vi "MM9.SetStatus.vi"(0 "i ref in":refnum<vi>, 1 "MMStatusSuccess":T1, 2 "MMStatusFail":T1, 3 "ms timeout (10000)":i32=10000, 5 "error in (no error)":errorcluster) -> (14 "i ref out":refnum<vi>, 16 "StatusText":string, 17 "timed out":bool, 19 "error out":errorcluster)   [LabVIEW 2014, in "MM9.lvlib"]
doc: "Sets the status of the measurement."
uses:
  MM9.lvlib
  MM9.status.ctl
  CS_Core/CSSystem/CoreLib/CoreLib.lvlib
  CSlibraries-extern/DimLVEvent/LVDimInterface/LVDimInterface.lvlib
panel:
  in  "MMStatus":T1=enum."config"
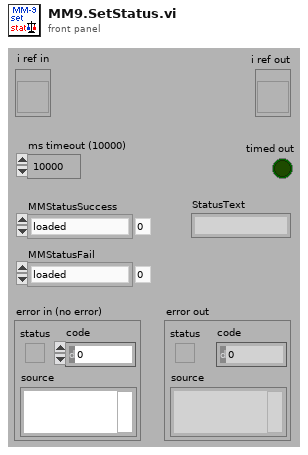
[diagram p1: front panel]
types:
  T1 = typedef "MM9.lvlib/MM9.status.ctl" = enum16{"loaded", "load_error", "config", "config_error", "init", "init_error", "data_reset", "data_reset_error", "running", "start_error", "run_error", "abort_requested", "aborted", "stop_requested", "stopped", "stop_error", "Connected", "NOTConnected"}
  T2 = typedef "MM9.lvlib/MM9.i attribute.ctl" = cluster{"UsedObjs":string[], "ActScanStep":i32[], "AbortRequest":bool, "StopRequest":bool, "# cycles":i32, "Connected":bool, "MMStatus":T1, "# data":i32, "DIMServices":cluster{"MM6StatusString":string, "MM6StatusID":i32, "discArchiver":string, "discArchiverID":i32, "eventBuilder":string, "eventBuilderID":i32, "GUIIDString":string, "GUIIDStringID":i32}, "dataFile":string, "PGRunning":T3, "ConfigData":T4, "ExtraDataSets":T19}
  T3 = typedef "PPG_ABC.lvlib/PPG_ABC.PG_Running.ctl" = i32
  T4 = typedef "LEBITDefs9.lvlib/LEBITDefs.ConfigData.ctl" = cluster{"GenConfig":T5, "Configs":T7[]}
  T5 = typedef "LEBITDefs9.lvlib/LEBITDefs.GenConfig.ctl" = cluster{"Mode":i32, "Logs":T6[]}
  T6 = typedef "LEBITDefs9.lvlib/LEBITDefs.Log.ctl" = cluster{"Name":string, "FctName":string, "Special":string}
  T7 = typedef "LEBITDefs9.lvlib/LEBITDefs.OneConfig.ctl" = cluster{"MCA":T8, "Timing":T9, "Scans":T12[], "FreqDevs":T13[], "CleanDev":T14, "NrCycles":i32, "Specials":T16[], "Delays":T17[], "DAC":T18}
  T8 = typedef "LEBITDefs9.lvlib/LEBITDefs.MCA.ctl" = cluster{"Name":string, "Address":string, "NrChannels":i32, "Gate":i32, "NrPipse":i32, "AcqDelay":i32}
  T9 = typedef "LEBITDefs9.lvlib/LEBITDefs.Timing.ctl" = cluster{"TimeTables":cluster{"TimeTable":T10}[], "Memories":T11[], "ScanX":string, "ScanY":string}
  T10 = typedef "LEBITDefs9.lvlib/LEBITDefs.Timetable.ctl" = dbl[]
  T11 = typedef "LEBITDefs9.lvlib/LEBITDefs.Memory.ctl" = cluster{"Device":string, "ExtTrig":bool, "TT2Use":i32, "PatternTable":string[]}
  T12 = typedef "LEBITDefs9.lvlib/LEBITDefs.ScanDev.ctl" = cluster{"Name":string, "FctName":string, "Values":dbl[], "NrScanVals":i32, "Special":string}
  T13 = typedef "LEBITDefs9.lvlib/LEBITDefs.FreqDev.ctl" = cluster{"Name":string, "Amp":dbl, "CenterFreq":dbl, "Time":dbl}
  T14 = typedef "LEBITDefs9.lvlib/LEBITDefs.CleanDev.ctl" = cluster{"Name":string, "CleanData":T15[]}
  T15 = typedef "LEBITDefs9.lvlib/LEBITDefs.CleanDataType.ctl" = cluster{"Amp":dbl, "Center":dbl, "Plus":dbl, "Minus":dbl, "Time":dbl}
  T16 = typedef "LEBITDefs9.lvlib/LEBITDefs.Special.ctl" = cluster{"Name":string, "FctName":string, "VerySpecial":string, "Data":dbl}
  T17 = typedef "LEBITDefs9.lvlib/LEBITDefs.Delay.ctl" = cluster{"Name":string, "Delay":dbl}
  T18 = typedef "LEBITDefs9.lvlib/LEBITDefs.DAC.ctl" = cluster{"Name":string, "Step1":i32, "Step2":i32}
  T19 = typedef "LEBITDefs9.lvlib/LEBITDefs.ExtraData.ctl" = cluster{"Ions":cluster{"ExcitIonMass":string, "ExcitIonCharge":i32, "CleanIons":cluster{"CleanIonMass":string, "CleanIonCharge":i32}[]}, "TimingDescription":cluster{"TimeTableDescription":cluster{"Times":string[]}[], "PatternTableDescription":cluster{"Pattern":string[]}[]}, "ScanUnits":string[]}[]
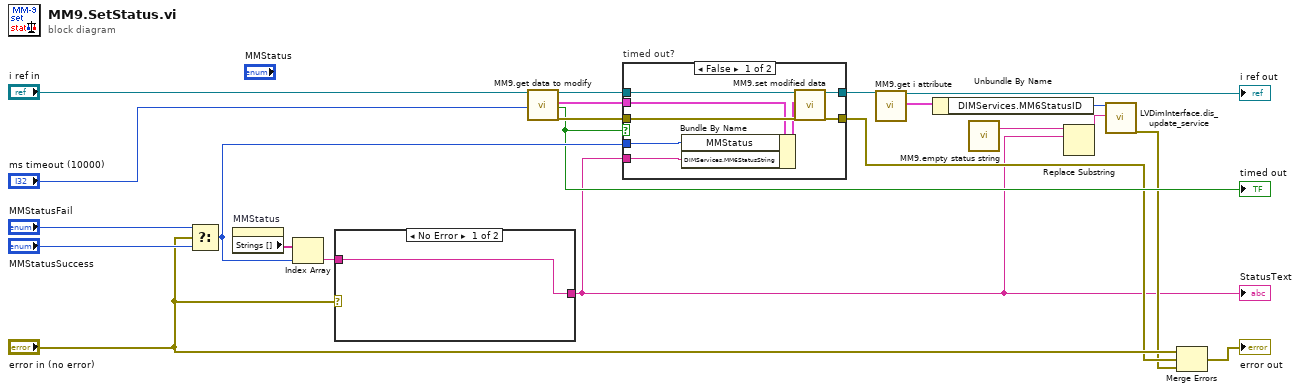
[diagram p0: block diagram]
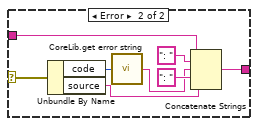
[diagram p3: hidden frame]
diagram:
  n1 = Select(t="MMStatusFail", s="error in (no error)", f="MMStatusSuccess") -> (s? t:f=w16:T1)
  n2 = property on="MMStatus" class="Enum (strict)"() -> ("Strings []"=w15:string[])  [unwired: 2 in, 2 out]
  n3 = Index Array(array=w15, index=w16) -> (element=w14:string)
  n4 = case shown="No Error" "error in (no error)" {
    selector: "error in (no error)" -> [_ w31]
    tunnel: [w23 w27] -> w3
    tunnel: w14 -> [w23 w24]
    frame No Error {
    }
    frame Error {
      n5 = Unbundle By Name(w31) -> ("code"=w30:i32, "source"=w28:string)
      n6 = call "CoreLib.get error string.vi"("Error Code"=w30) -> ("Error String"=w26:string)
      n7 = Concatenate Strings(w24, ": " ("string"), w26, ": " ("string"), w28) -> (w27:string)
    }
  }
  "StatusText" <- w3
  n8 = call "MM9.get data to modify.vi"("i ref in"="i ref in", "ms timeout (10000)"="ms timeout (10000)") -> ("i ref out"=w22:refnum<vi>, "i attribute"=w20:T2, "timed out"=w13:bool, "error out"=w21:errorcluster)  [unwired: 14 in]
  "timed out" <- w13
  n9 = case "timed out?" shown="False" w13 {
    tunnel: w22 -> [w38 w41]
    tunnel: [w39 w41] -> w8
    tunnel: w21 -> [w37 w40]
    tunnel: w20 -> [w36 _]
    tunnel: w16 -> [w34 _]
    tunnel: [w33 w40] -> w11
    tunnel: w3 -> [w32 _]
    frame False {
      n10 = Bundle By Name(cluster=w36, "MMStatus"=w34, "DIMServices.MM6StatusString"=w32) -> (w35:T2)
      n11 = call "MM9.set modified data.vi"("i ref in"=w38, "i attribute"=w35, "error in (no error)"=w37) -> ("i ref out"=w39:refnum<vi>, "error out"=w33:errorcluster)  [unwired: 15 in]
    }
    frame True {
    }
  }
  n12 = call "MM9.get i attribute.vi"("i ref in"=w8) -> ("i ref out"=→"i ref out":refnum<vi>, "i attribute"=w7:T2)  [unwired: 16 in, 1 out]
  n13 = Unbundle By Name(w7) -> ("DIMServices.MM6StatusID"=w6:i32)
  n14 = call "MM9.empty status string.vi"() -> ("String"=w5:string)
  n15 = Replace Substring(4:w3, 5:w5) -> (1:w4:string)  [unwired: 2 in, 1 out]
  n16 = call "LVDimInterface.dis_update_service.vi"("my_serviceID"=w6, "data"=w4) -> ("error out"=w9:errorcluster)  [unwired: 15 in, 2 out]
  n17 = Merge Errors("error in (no error)", w11, w9) -> (→"error out":errorcluster)
